vi "Multiple U3 with Multiple AIN Parallel.vi"() -> ()   [LabVIEW 2021]
panel:
  in  "Collect First n Channels From Each":u32=3
  out "All Readings":dbl[](array[numeric]) format="%.6f"
  in  "Device B Local ID":i32=2
  out "Readings B":dbl[](array[numeric]) format="%.6f"
  out "Error Message B":string
  in  "Device A Local ID":i32=1
  out "Readings A":dbl[](array[numeric]) format="%.6f"
  in  "stop":bool
  in  "Interval (ms)":u32=500
  out "Error Message A":string
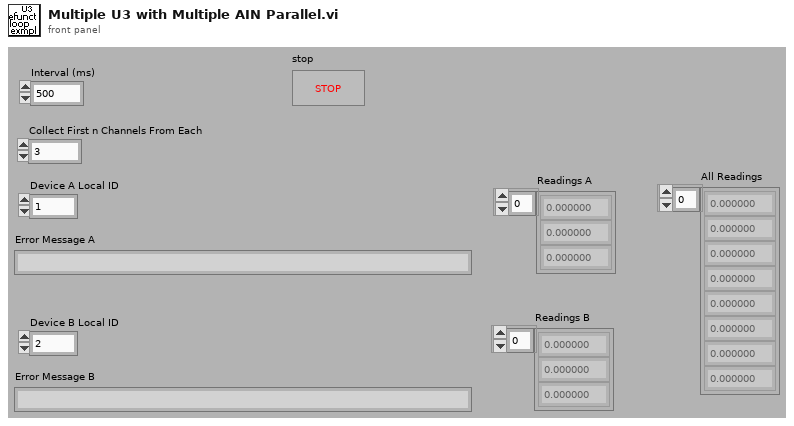
[diagram p1: front panel]
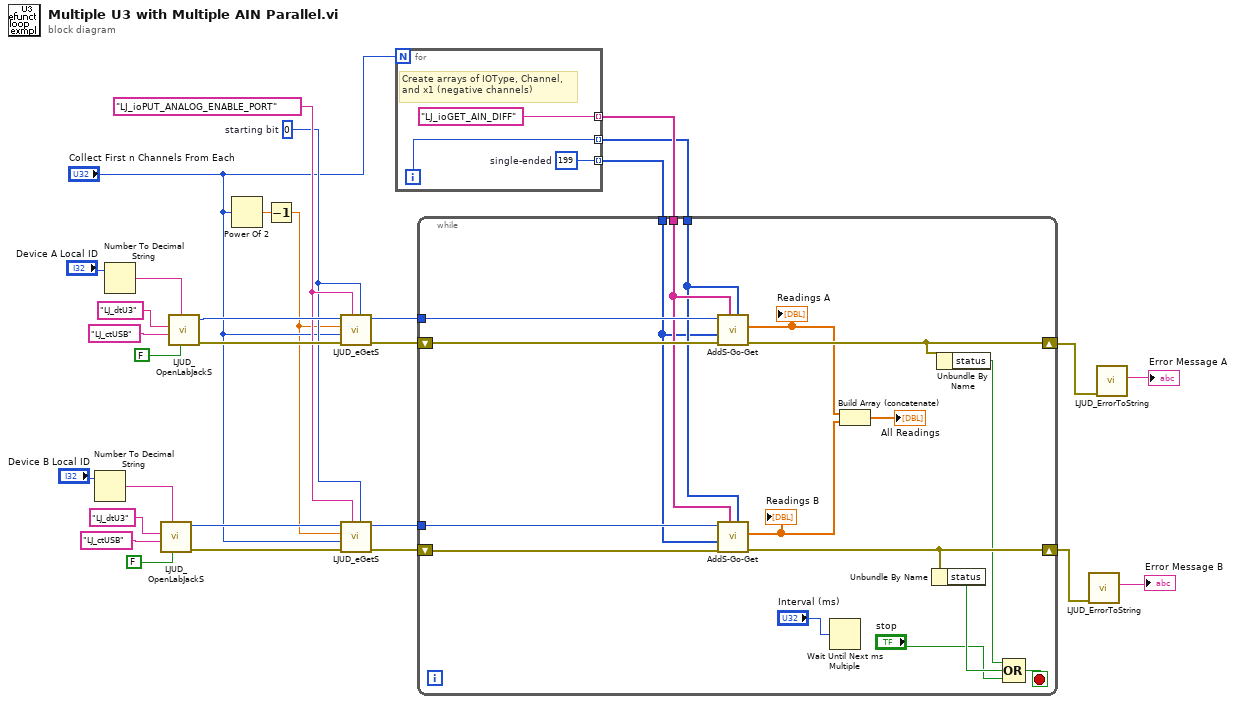
[diagram p0: block diagram]
diagram:
  w7 = "LJ_ioPUT_ANALOG_ENABLE_PORT" ("IOType")
  w6 = 0  # starting bit
  n1 = Number To Decimal String(number="Device B Local ID") -> (decimal integer string=w15:string)  [unwired: 1 in]
  n2 = Number To Decimal String(number="Device A Local ID") -> (decimal integer string=w16:string)  [unwired: 1 in]
  n3 = call "LJUD_OpenLabJackS.vi"("FirstFound"=FALSE, "Address"=w15, "ConnectionType"="LJ_ctUSB", "DeviceType"="LJ_dtU3") -> ("error out"=w14:errorcluster, "Handle"=w12:i32)  [unwired: 5 in, 1 out]
  n4 = call "LJUD_OpenLabJackS.vi"("FirstFound"=FALSE, "Address"=w16, "ConnectionType"="LJ_ctUSB", "DeviceType"="LJ_dtU3") -> ("error out"=w22:errorcluster, "Handle"=w20:i32)  [unwired: 5 in, 1 out]
  n5 = Power Of 2(x="Collect First n Channels From Each") -> (2^x=w2:dbl)
  n6 = Decrement(x=w2) -> (x-1=w1:dbl)
  n7 = call "LJUD_eGetS.vi"("Channel"=w6, "IOType"=w7, "error in"=w22, "x1"="Collect First n Channels From Each", "Value Write"=w1, "Handle In"=w20) -> ("error out"=w21:errorcluster, "Handle Out"=w19:i32)  [unwired: 3 in, 1 out]
  n8 = call "LJUD_eGetS.vi"("Channel"=w6, "IOType"=w7, "error in"=w14, "x1"="Collect First n Channels From Each", "Value Write"=w1, "Handle In"=w12) -> ("error out"=w13:errorcluster, "Handle Out"=w11:i32)  [unwired: 3 in, 1 out]
  n9 = for {
    N: "Collect First n Channels From Each" -> [_]
    tunnel: ["LJ_ioGET_AIN_DIFF" ("IOType")] -> w10 mode=indexing
    tunnel: [w32] -> w9 mode=indexing
    tunnel: [w31] -> w8 mode=indexing
    i -> [w32]
    w31 = 199  # single-ended
    # "Create arrays of IOType, Channel,\nand x1 (negative channels)"
  }
  n10 = while {
    tunnel: w8 -> [w37]
    tunnel: w9 -> [w38]
    tunnel: w10 -> [w39]
    tunnel: w11 -> [w42]
    tunnel: w19 -> [w43]
    shift-left: w21 -> [w40]
    shift-right: [w46] -> w23
    shift-left: w13 -> [w41]
    shift-right: [w49] -> w28
    stop <- w44 stop-if-true
    n11 = call "AddS-Go-Get.vi"("Channels"=w38, "IOTypes"=w39, "error in"=w40, "x1"=w37, "Handle In"=w43) -> ("error out"=w46:errorcluster, "Values Read"=w36:dbl[])  [unwired: 4 in, 1 out]
    "Readings A" <- w36
    n12 = call "AddS-Go-Get.vi"("Channels"=w38, "IOTypes"=w39, "error in"=w41, "x1"=w37, "Handle In"=w42) -> ("error out"=w49:errorcluster, "Values Read"=w35:dbl[])  [unwired: 4 in, 1 out]
    "Readings B" <- w35
    n13 = Wait Until Next ms Multiple(millisecond multiple="Interval (ms)") -> ()  [unwired: 1 out]
    n14 = Build Array (concatenate)(w36, w35) -> (→"All Readings":dbl[])
    n15 = Unbundle By Name(w49) -> ("status"=w48:bool)
    n16 = Unbundle By Name(w46) -> ("status"=w45:bool)
    n17 = Compound Arithmetic op=OR(w45, w48, "stop") -> (w44:bool)
  }
  n18 = call "LJUD_ErrorToString.vi"("error in"=w28) -> ("String"=→"Error Message B":string)  [unwired: 10 in]
  n19 = call "LJUD_ErrorToString.vi"("error in"=w23) -> ("String"=→"Error Message A":string)  [unwired: 10 in]
